vi "rc_interrupt_Init.vi"(8 "error in (no error)":errorcluster) -> (0 "error out":errorcluster, 3 "function return":i32)   [LabVIEW 2014, in "Interrupt.lvlib"]
doc: "int Init();"
uses:
  Interrupt.lvlib
  <vilib>/wsapi/NI_WebServices.lvlib
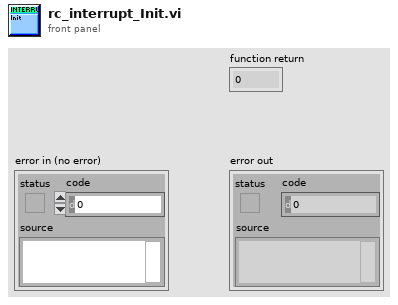
[diagram p1: front panel]
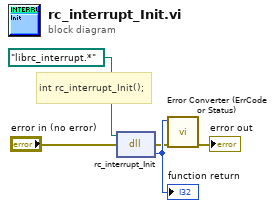
[diagram p0: block diagram]
diagram:
  # "int rc_interrupt_Init();"
  n1 = dll-call lib="C:/Users/ktalke/Documents/Jessie Build/Interrupt/Interrupt.so" fn="rc_interrupt_Init"(path in=path "librc_interrupt.*", error in="error in (no error)") -> (error out=w3:errorcluster, "return type"=w5:i32)  [unwired: 1 in, 1 out]
  "function return" <- w5
  n2 = call <vilib>:"Error Converter (ErrCode or Status).vi"("error in (no error)"=w3, "error code"=w5) -> ("error out"=→"error out":errorcluster)  [unwired: 9 in]
